vi "Test Move Straight.vi"() -> ()   [LabVIEW 2016]
panel:
  in  "Angle":dbl
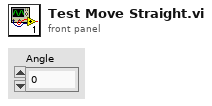
[diagram p1: front panel]
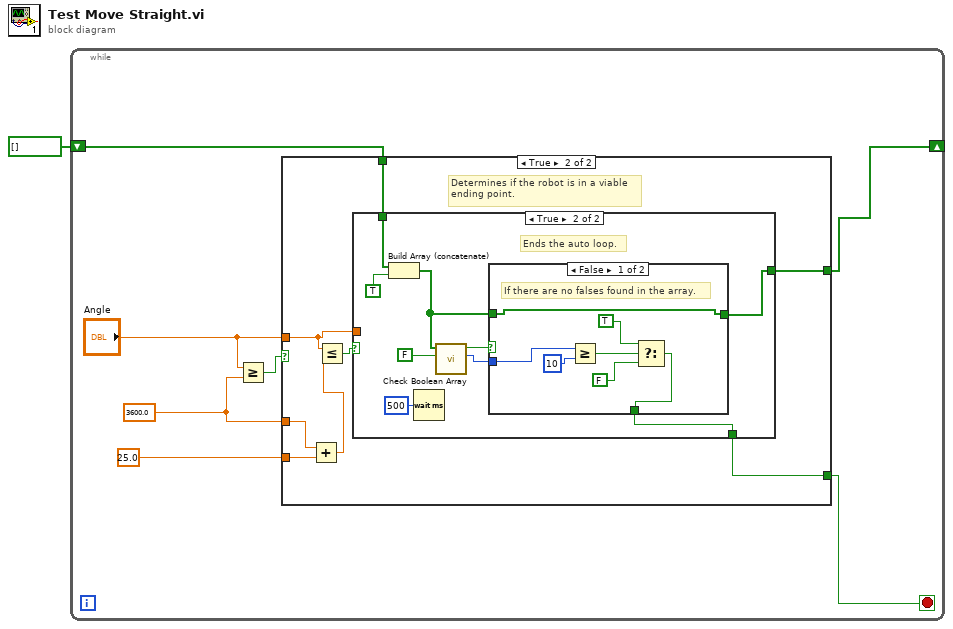
[diagram p0: block diagram]
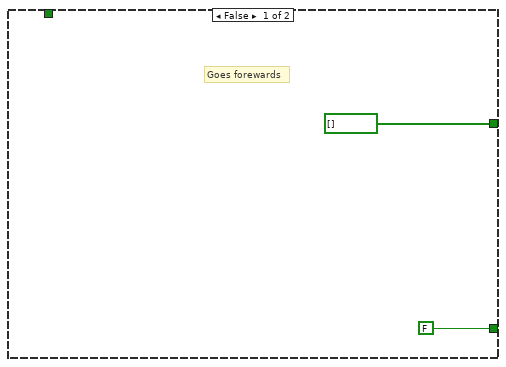
[diagram p2: hidden frame]
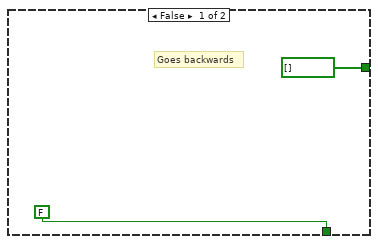
[diagram p3: hidden frame]
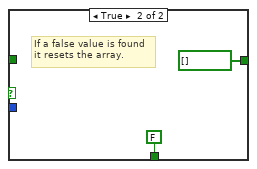
[diagram p4: hidden frame]
diagram:
  n1 = while {
    shift-right: [w3] -> _
    shift-left: bool[] [] -> [w2]
    stop <- w5 stop-if-true
    w7 = 3600.0 ("Encoder Position")
    n2 = Greater Or Equal?(x="Angle", y=w7) -> (x >= y?=w4:bool)
    n3 = case shown="True" w4 {
      tunnel: "Angle" -> [_ w13]
      tunnel: w7 -> [_ w17]
      tunnel: [FALSE w15] -> w5
      tunnel: [bool[] [] w14] -> w3
      tunnel: 25.0 ("y") -> [_ w12]
      tunnel: w2 -> [_ w11]
      frame False {
        # "Goes forewards"
      }
      frame True {
        # "Determines if the robot is in a viable\nending point."
        n4 = Add(x=w17, y=w12) -> (x+y=w16:dbl)
        n5 = Less Or Equal?(x=w13, y=w16) -> (x <= y?=w18:bool)
        n6 = case shown="True" w18 {
          tunnel: w13 -> [_ _]
          tunnel: [FALSE w22] -> w15
          tunnel: [bool[] [] w24] -> w14
          tunnel: w11 -> [_ w21]
          frame False {
            # "Goes backwards"
          }
          frame True {
            # "Ends the auto loop."
            n7 = Build Array (concatenate)(w21, TRUE) -> (w25:bool[])
            n8 = Wait (ms)(milliseconds to wait=u32 500) -> ()  [unwired: 1 out]
            n9 = call "Check Boolean Array.vi"("Search For"=FALSE, "Array"=w25) -> ("Array Size"=w23:i32, "Found"=w26:bool)  [unwired: 8 in]
            n10 = case shown="False" w26 {
              tunnel: w25 -> [w31 _]
              tunnel: [w31 bool[] []] -> w24
              tunnel: w23 -> [w30 _]
              tunnel: [w32 FALSE ("Search For")] -> w22
              frame False {
                # "If there are no falses found in the array."
                n11 = Greater Or Equal?(x=w30, y=10) -> (x >= y?=w33:bool)
                n12 = Select(t=TRUE, s=w33, f=FALSE ("Search For")) -> (s? t:f=w32:bool)
              }
              frame True {
                # "If a false value is found\nit resets the array."
              }
            }
          }
        }
      }
    }
  }
